vi "Stop Driving.vi"(7 "Description":string, 8 "Command Info In":T1) -> (0 "Command Info Out":T1)   [LabVIEW 2017]
doc: "Zero the drive motors, making the robot stationary."
uses:
  <vilib>/Rock Robotics/WPI/Framework/Command Status Info.ctl
  <vilib>/Rock Robotics/WPI/Framework/Completion Status.ctl
  <vilib>/Rock Robotics/WPI/Framework/Completion Notifier.ctl
  Implementation/Drive Setpoints.ctl
  Implementation/Drive Operations.ctl
  Shared/RobotNeededPathData.ctl
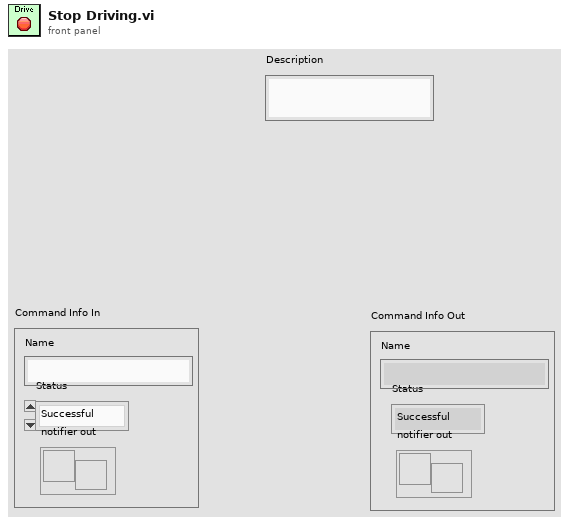
[diagram p1: front panel]
types:
  T1 = typedef "Command Status Info.ctl" = cluster{"Name":string, "Status":T2, "notifier out":T3}
  T2 = typedef "Completion Status.ctl" = enum16{"Successful", "Aborted", "Incomplete"}
  T3 = typedef "Completion Notifier.ctl" = refnum<notifier>
  T4 = typedef "Drive Setpoints.ctl" = cluster{"Operation":T5, "Left Speed":dbl, "Right Speed":dbl, "Duration":dbl, "Speed":dbl, "Start Angle":dbl, "Target Angle":dbl, "Distance (inch)":dbl, "Start Point (inch)":dbl, "RobotNeededPathData":T6}
  T5 = typedef "Drive Operations.ctl" = enum16{"Reserve", "Read Current", "Immediate", "Drive for Time", "Drive for Distance", "Turn to Angle", "Arc Turn", "Drive Path"}
  T6 = typedef "RobotNeededPathData.ctl" = cluster{"Path":cluster{dbl, dbl}[], "MaxVel":dbl, "MaxAccel":dbl, "Backwards?":bool, "PointSpacing":dbl, "LookaheadDist":dbl, "Speed/Curve":dbl, "SlowDistanceAtEnd":dbl, "SlowSpeed":dbl}
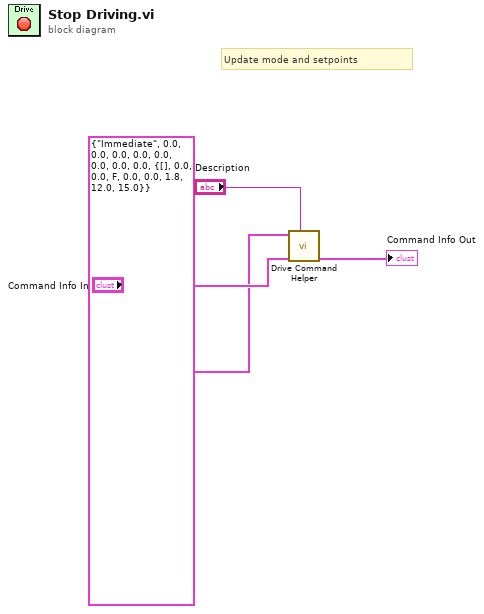
[diagram p0: block diagram]
diagram:
  # "Update mode and setpoints"
  n1 = call "Drive Command Helper.vi"("Description"="Description", "Command Info In"="Command Info In", "SubSystem Data"=T4 {"Operation"=enum."Immediate", "Left Speed"=0.0, "Right Speed"=0.0, "Duration"=0.0, "Speed"=0.0, "Start Angle"=0.0, "Target Angle"=0.0, "Distance (inch)"=0.0, "Start Point (inch)"=0.0, "RobotNeededPathData"={"Path"=[], "MaxVel"=0.0, "MaxAccel"=0.0, "Backwards?"=FALSE, "PointSpacing"=0.0, "LookaheadDist"=0.0, "Speed/Curve"=1.8, "SlowDistanceAtEnd"=12.0, "SlowSpeed"=15.0}}) -> ("Command Info Out"=→"Command Info Out":T1)  [unwired: 6 in, 2 out]
